vi "Write Textual.vi"(8 "error in (no error)":errorcluster, 10 "Textual":bool, 11 "TCP Writer in":refnum<class "TCP Writer.lvclass">) -> (0 "error out":errorcluster, 3 "TCP Writer out":refnum<class "TCP Writer.lvclass">)   [LabVIEW 2020, in "TALOS.lvlib" / "TCP Writer.lvlib" / "TCP Writer.lvclass"]
uses:
  TCP Writer.lvclass
  TCP Writer.lvclass/TCP Writer.ctl
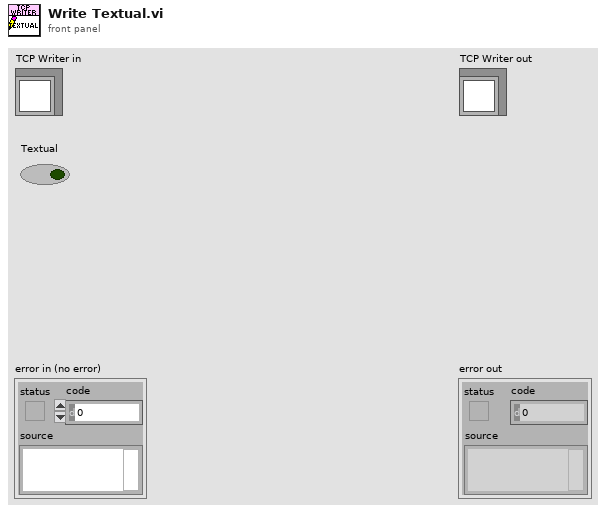
[diagram p1: front panel]
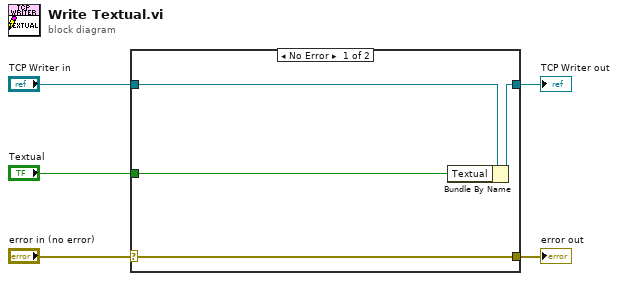
[diagram p0: block diagram]
diagram:
  n1 = case shown="No Error" "error in (no error)" {
    selector: "error in (no error)" -> [w9 w10]
    tunnel: [w9 w10] -> w4
    tunnel: [w7 w11] -> w2
    tunnel: "TCP Writer in" -> [w8 w11]
    tunnel: "Textual" -> [w6 _]
    frame No Error {
      n2 = Bundle By Name(cluster=w8, "Textual"=w6) -> (w7:refnum<class "TCP Writer.lvclass">)
    }
    frame Error {
    }
  }
  "error out" <- w4
  "TCP Writer out" <- w2
